vi "write_config_settings.vi"() -> ()   [LabVIEW 2011]
doc: "Illustrates how to create and write a configuration settings file.\n\nInstructions:\nEnter values in the controls on the front panel then click on the Run Arrow.\nTo read the file, run Read Configuration Settings File.vi located in the file\\config.llb."
uses:
  <vilib>/Utility/config.llb/Write Key (Boolean).vi
  <vilib>/Utility/config.llb/Write Key (Double).vi
  <vilib>/Utility/config.llb/Write Key (Path).vi
  <vilib>/Utility/config.llb/Write Key (String).vi
  <vilib>/Utility/config.llb/NI_LVConfig.lvlib
panel:
  in  "String 2":string="This string contains no unprintable characters. Set the Write Raw String input of Write Key (String) to TRUE to write it to file without escaping the string."
  in  "String 1":string="This string contains unprintable characters,\nspecifically the linefeed (x0A) character, that\nmust be \"escaped\" before writing them to\nfile. The Configuration File VIs do this\nescaping by default.  Set the Write Raw String input\nof Write Key (String) to TRUE to write it to file without\nescaping the string."
  in  "Boolean":bool
  in  "Numeric":dbl=2.0 format="%0.2f"
  in  "Path Value":path=path "C:/My Path Name"
  # "Instructions:\nEnter values in the controls below, then click on the Run arrow.  The VI will write these values into the selected configuration settings file.\n\nTo read the file, run Read Configuration Settings File.vi located in the file\\config.llb."
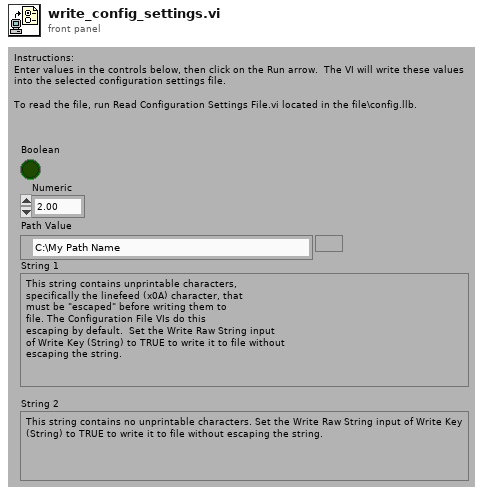
[diagram p1: front panel]
types:
  T1 = typedef "NI_LVConfig.lvlib/Config Data RefNum.ctl" = refnum<k1>
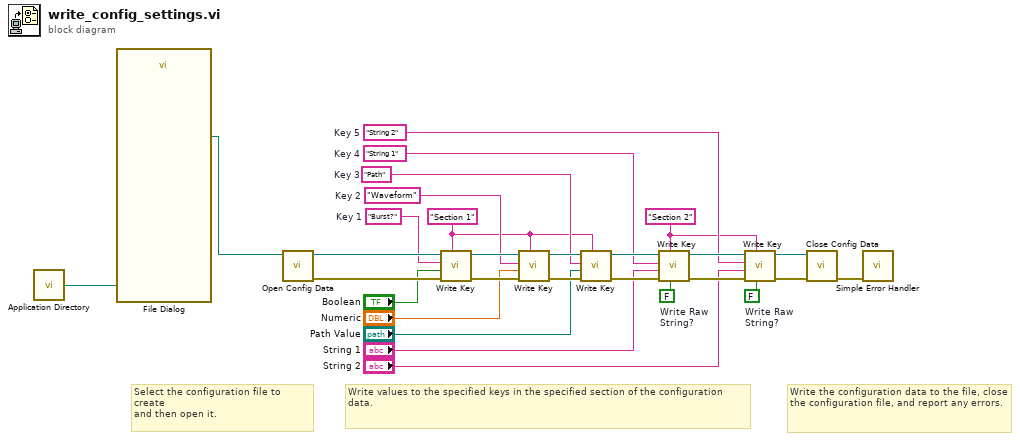
[diagram p0: block diagram]
diagram:
  w3 = FALSE  # Write Raw String?
  w4 = FALSE  # Write Raw String?
  w13 = "String 2"  # Key 5
  w14 = "String 1"  # Key 4
  w15 = "Path"  # Key 3
  w16 = "Waveform"  # Key 2
  w17 = "Burst?"  # Key 1
  w8 = "Section 2"
  w9 = "Section 1"
  # "Write the configuration data to the file, close the configuration file, and report any errors."
  # "Write values to the specified keys in the specified section of the configuration data."
  # "Select the configuration file to create\nand then open it."
  n1 = call <vilib>:"Application Directory.vi"() -> ("Application Directory"=w1:path)
  n2 = call "File Dialog"("start path"=w1) -> ("selected path"=w2:path)  [unwired: 11 in, 3 out]
  n3 = call <vilib>:"Open Config Data.vi"("configuration file path"=w2) -> ("error out"=w23:errorcluster, "refnum"=w29:T1)  [unwired: 2 in, 7 out]
  n4 = call-poly <vilib>:"Write Key.vi"("section"=w9, "error in (no error)"=w23, "value"="Boolean", "key"=w17, "refnum"=w29) -> ("error out"=w22:errorcluster, "refnum out"=w28:T1)  [unwired: 5 out]
  n5 = call-poly <vilib>:"Write Key.vi"("section"=w9, "error in (no error)"=w22, "value"="Numeric", "key"=w16, "refnum"=w28) -> ("error out"=w21:errorcluster, "refnum out"=w27:T1)  [unwired: 3 in, 2 out]
  n6 = call-poly <vilib>:"Write Key.vi"("section"=w9, "error in (no error)"=w21, "value"="Path Value", "key"=w15, "refnum"=w27) -> ("error out"=w20:errorcluster, "refnum out"=w26:T1)  [unwired: 5 out]
  n7 = call-poly <vilib>:"Write Key.vi"("write raw string? (F)"=w3, "section"=w8, "error in (no error)"=w20, "value"="String 1", "key"=w14, "refnum"=w26) -> ("error out"=w19:errorcluster, "refnum out"=w25:T1)  [unwired: 4 out]
  n8 = call-poly <vilib>:"Write Key.vi"("write raw string? (F)"=w4, "section"=w8, "error in (no error)"=w19, "value"="String 2", "key"=w13, "refnum"=w25) -> ("error out"=w18:errorcluster, "refnum out"=w24:T1)  [unwired: 4 out]
  n9 = call <vilib>:"Close Config Data.vi"("error in (no error)"=w18, "refnum"=w24) -> ("error out"=w10:errorcluster)  [unwired: 1 in, 8 out]
  n10 = call <vilib>:"Simple Error Handler.vi"("error in (no error)"=w10) -> ()  [unwired: 1 in, 8 out]
